vi "Read Replot request.vi"(8 "error in (no error)":errorcluster, 11 "Plot in":refnum<class "Plot.lvclass">) -> (0 "error out":errorcluster, 2 "Replot request":bool, 3 "Plot out":refnum<class "Plot.lvclass">)   [LabVIEW 2019, in "Plot.lvclass"]
uses:
  Plot.lvclass
  Plot.lvclass/Plot.ctl
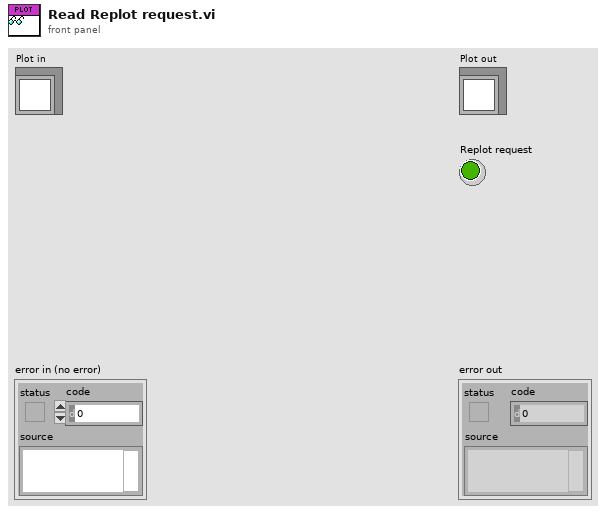
[diagram p1: front panel]
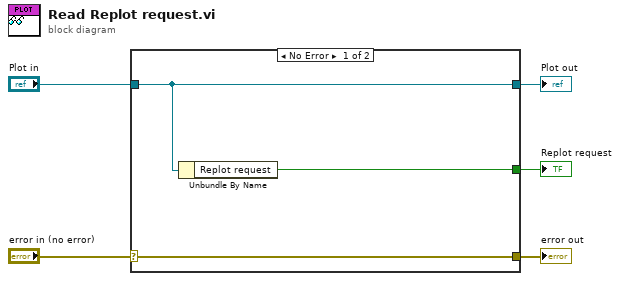
[diagram p0: block diagram]
diagram:
  n1 = case shown="No Error" "error in (no error)" {
    selector: "error in (no error)" -> [w8 w9]
    tunnel: [w8 w9] -> w4
    tunnel: [w7 w10] -> w2
    tunnel: "Plot in" -> [w7 w10]
    tunnel: [w6 _] -> w1
    frame No Error {
      n2 = Unbundle By Name(w7) -> ("Replot request"=w6:bool)
    }
    frame Error {
    }
  }
  "error out" <- w4
  "Plot out" <- w2
  "Replot request" <- w1
